vi "gxml_TypeCheck.vi"(8 "error in":errorcluster, 9 "Type Enum":T1, 10 "XML Item Attributes":string, 11 "Item Name":string) -> (0 "error out":errorcluster)   [LabVIEW 2011, in "Third Party VIs.lvlib" / "GXML.lvlib"]
uses:
  <vilib>/Utility/VariantDataType/Type.ctl
  <vilib>/regexp/Match Regular Expression.xnode
  GXML.lvlib
  <vilib>/Utility/VariantDataType/VariantType.lvlib
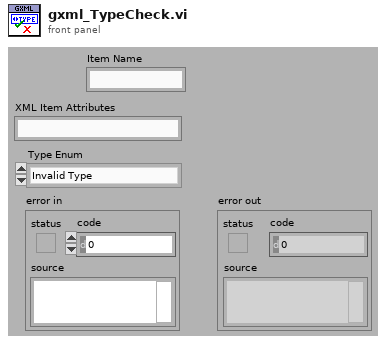
[diagram p1: front panel]
types:
  T1 = typedef "VariantType.lvlib/Type.ctl" = enum8{"Invalid Type", "Void", "I8", "I16", "I32", "I64", "U8", "U16", "U32", "U64", "Single Float", "Double Float", "Extended Float", "Single Complex", "Double Complex", "Extended Complex", "Enum U8", "Enum U16", "Enum U32", "Enum U64", "Single Float With Unit", "Double Float With Unit", "Extended Float With Unit", "Single Complex with Unit", "Double Complex with Unit", "Extended Complex with Unit", "Boolean", "String", "Path", "Picture", "Tag", "Array", "Cluster", "Variant", "LV Variant", "Waveform", "Timestamp", "Digital Waveform", "Digital Data", "ExpressData", "Refnum", "External Data", "VI", "Poly VI", "LabVIEW Class Instance", "Fixed Point"}
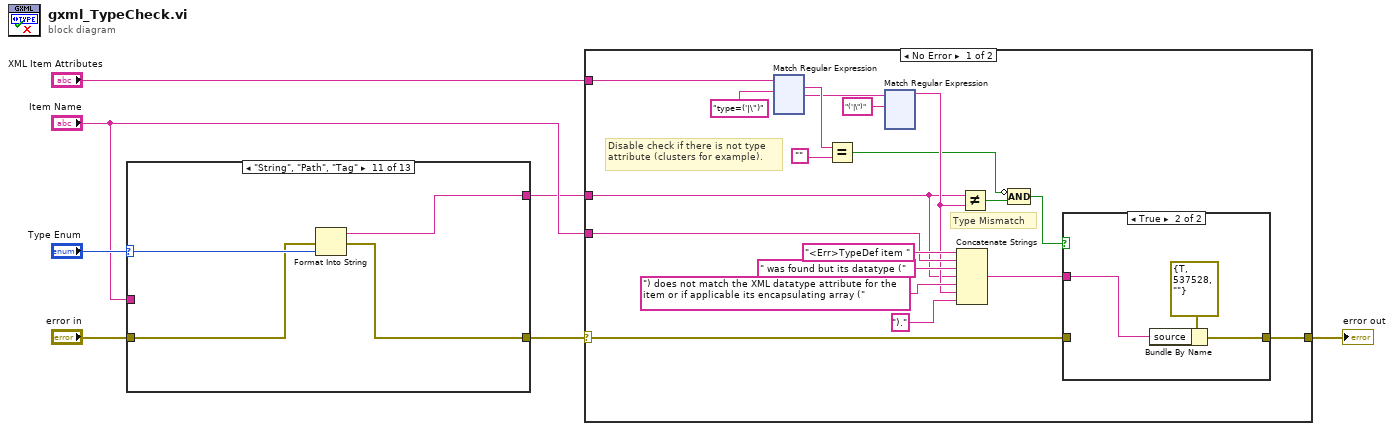
[diagram p0: block diagram]
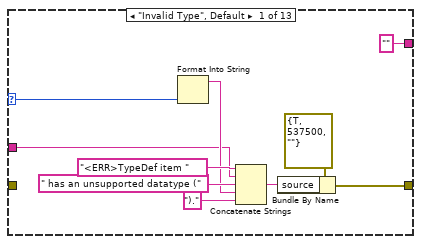
[diagram p2: hidden frame]
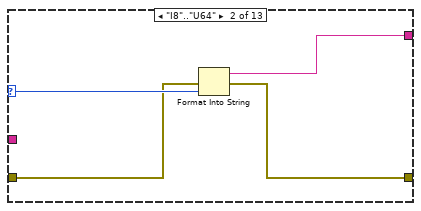
[diagram p3: hidden frame]
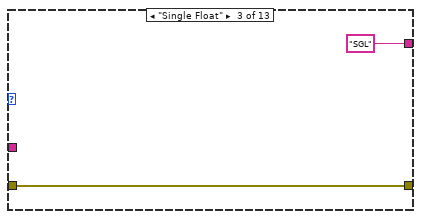
[diagram p4: hidden frame]
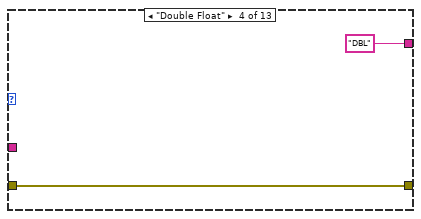
[diagram p5: hidden frame]
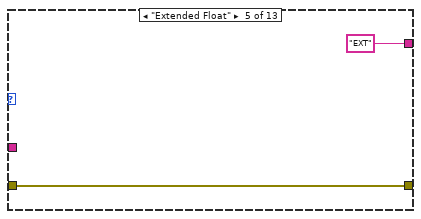
[diagram p6: hidden frame]
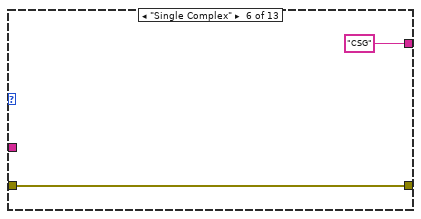
[diagram p7: hidden frame]
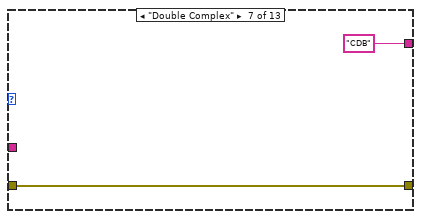
[diagram p8: hidden frame]
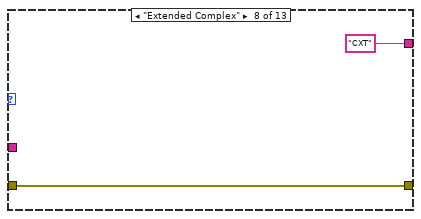
[diagram p9: hidden frame]
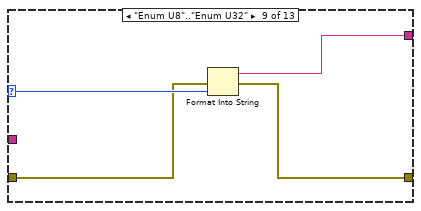
[diagram p10: hidden frame]
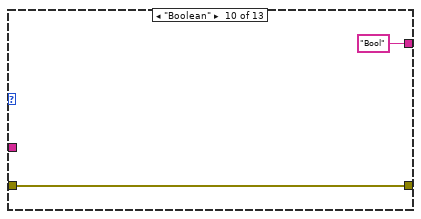
[diagram p11: hidden frame]
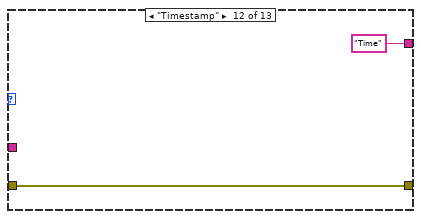
[diagram p12: hidden frame]
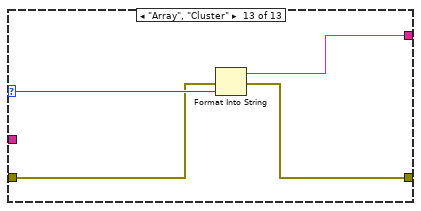
[diagram p13: hidden frame]
diagram:
  n1 = case shown="\"String\", \"Path\", \"Tag\"" "Type Enum" {
    selector: "Type Enum" -> [w9 w21 _ _ _ _ _ _ w37 _ w43 _ w49]
    tunnel: ["" ("y") w20 "SGL" ("y") "DBL" ("y") "EXT" ("y") "CSG" ("y") "CDB" ("y") "CXT" ("y") w36 "Bool" ("y") w42 "Time" ("y") w48] -> w1
    tunnel: "error in" -> [_ w19 w22 w24 w26 w28 w30 w32 w35 w38 w41 w44 w47]
    tunnel: [w10 w18 w22 w24 w26 w28 w30 w32 w34 w38 w40 w44 w46] -> w5
    tunnel: "Item Name" -> [w8 _ _ _ _ _ _ _ _ _ _ _ _]
    frame "Invalid Type", Default {
      n2 = Format Into String(w9) -> (resulting string=w12:string)  [unwired: 3 in, 1 out]
      n3 = Concatenate Strings("<ERR>TypeDef item " ("Format String"), w8, " has an unsupported datatype (" ("Format String"), w12, ")." ("string")) -> (w16:string)
      n4 = Bundle By Name(cluster=errorcluster {"status"=TRUE, "code"=537500, "source"=""} ("error in"), "source"=w16) -> (w10:errorcluster)
    }
    frame "I8".."U64" {
      n5 = Format Into String(error in=w19, w21) -> (resulting string=w20:string, error out=w18:errorcluster)  [unwired: 2 in]
    }
    frame "Single Float" {
    }
    frame "Double Float" {
    }
    frame "Extended Float" {
    }
    frame "Single Complex" {
    }
    frame "Double Complex" {
    }
    frame "Extended Complex" {
    }
    frame "Enum U8".."Enum U32" {
      n6 = Format Into String(error in=w35, w37) -> (resulting string=w36:string, error out=w34:errorcluster)  [unwired: 2 in]
    }
    frame "Boolean" {
    }
    frame "String", "Path", "Tag" {
      n7 = Format Into String(error in=w41, w43) -> (resulting string=w42:string, error out=w40:errorcluster)  [unwired: 2 in]
    }
    frame "Timestamp" {
    }
    frame "Array", "Cluster" {
      n8 = Format Into String(error in=w47, w49) -> (resulting string=w48:string, error out=w46:errorcluster)  [unwired: 2 in]
    }
  }
  n9 = case shown="No Error" w5 {
    selector: w5 -> [w55 w295]
    tunnel: [w64 w295] -> w7
    tunnel: "Item Name" -> [w61 _]
    tunnel: w1 -> [w54 _]
    tunnel: "XML Item Attributes" -> [w51 _]
    frame No Error {
      # "Type Mismatch"
      # "Disable check if there is not type attribute (clusters for example)."
      n10 = xnode "Match Regular Expression"("input string"=w51, "regular expression"="type=('|\")") -> ("whole match"=w66:string, "after match"=w50:string)  [unwired: 4 in, 3 out]
      n11 = Equal?(x=w66, y="") -> (x = y?=w52:bool)
      n12 = xnode "Match Regular Expression"("input string"=w50, "regular expression"="('|\")") -> ("before match"=w58:string)  [unwired: 4 in, 4 out]
      n13 = Concatenate Strings("<Err>TypeDef item ", w61, " was found but its datatype (" ("string"), w54, ") does not match the XML datatype attribute for the item or if applicable its encapsulating array (" ("string"), w58, ")." ("string")) -> (w56:string)
      n14 = Not Equal?(x=w54, y=w58) -> (x != y?=w53:bool)
      n15 = Compound Arithmetic op=AND(invert w52, w53) -> (w63:bool)
      n16 = case shown="True" w63 {
        tunnel: [w291 w293] -> w64
        tunnel: w56 -> [_ w292]
        tunnel: w55 -> [w291 _]
        frame False {
        }
        frame True {
          n17 = Bundle By Name(cluster=errorcluster {"status"=TRUE, "code"=537528, "source"=""} ("error IO"), "source"=w292) -> (w293:errorcluster)
        }
      }
    }
    frame Error {
    }
  }
  "error out" <- w7
